vi "Compile - Tx Buffered Channel Refs.vi"(6 "Packet Name":string, 7 "Timestamp Present?":bool, 8 "error in (no error)":errorcluster, 11 "Item Ref in":T1 format="%.0x") -> (0 "error out":errorcluster, 3 "Item Ref out":T1 format="%.0x", 4 "Tx Ref Array":T2(array[cluster]) {"VS Refs" format="%.0x"})   [LabVIEW 2019, in "UDP-Custom-Device System Explorer.lvlib"]
uses:
  UDP-Custom-Device System Explorer.lvlib
  <vilib>/NI VeriStand/Custom Device API/Custom Device Item Ref.ctl
  Property Accessors/Tx Packet Accessors.lvlib
  <vilib>/NI VeriStand/Custom Device API/Custom Device API.lvlib
  Property Accessors/Buffered Data Packet.lvlib
  <vilib>/NI VeriStand/Custom Device Tools/Custom Device Utility Library/Custom Device Utility Library.lvlib
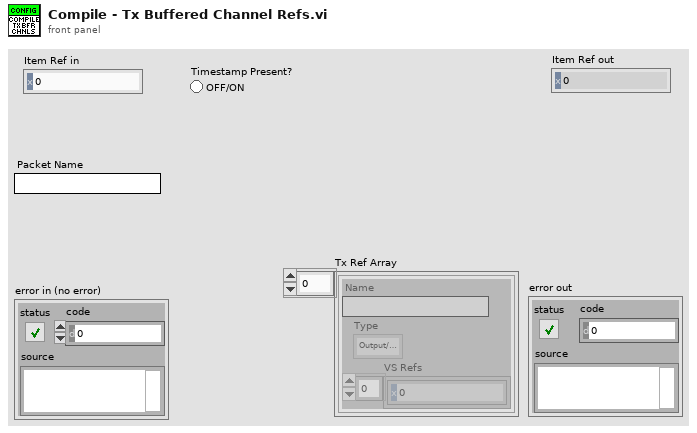
[diagram p1: front panel]
types:
  T1 = typedef "Custom Device API.lvlib/Custom Device Item Ref.ctl" = u64
  T2 = cluster{"Name":string, "Type":enum16{"Output/Write", "Input/Read", "Input/ReadWrite"}, "VS Refs":T1[]}[]
  T3 = cluster{"Name":string, "Type":enum16{"Output/Write", "Input/Read", "Input/ReadWrite"}, "VS Refs":T1[]}
  T4 = enum16{"Output/Write", "Input/Read", "Input/ReadWrite"}
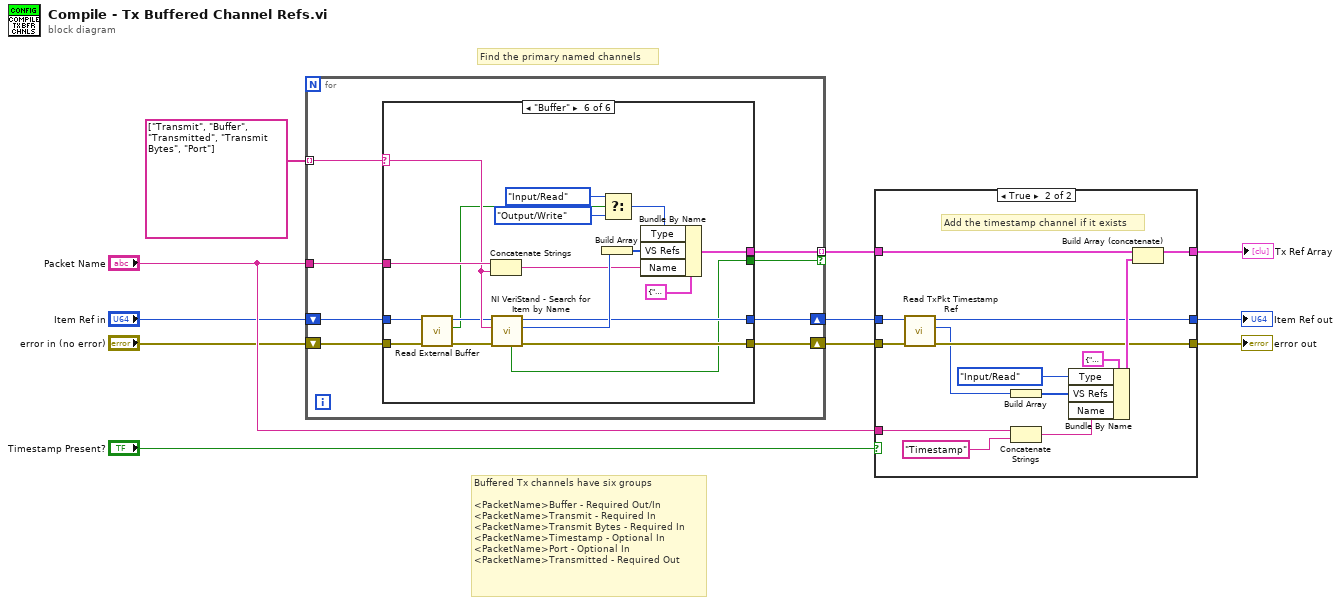
[diagram p0: block diagram]
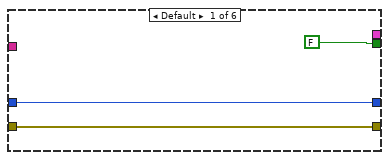
[diagram p3: hidden frame]
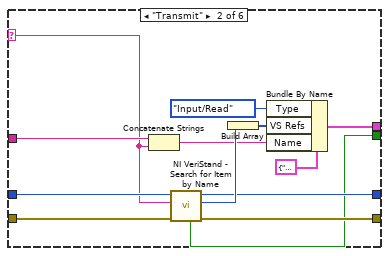
[diagram p4: hidden frame]
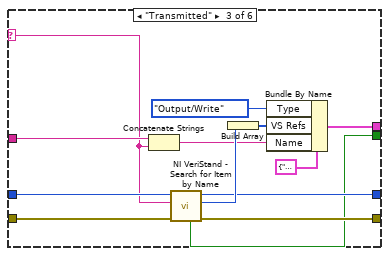
[diagram p5: hidden frame]
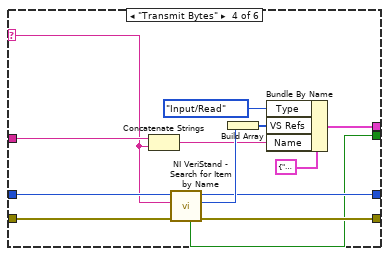
[diagram p6: hidden frame]
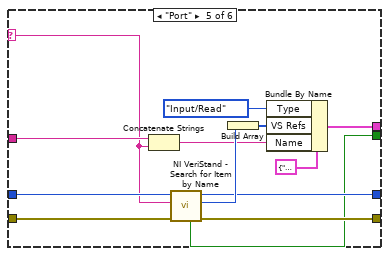
[diagram p7: hidden frame]
diagram:
  # "Find the primary named channels"
  # "Buffered Tx channels have six groups\n\n<PacketName>Buffer - Required Out/In\n<PacketName>Transmit - Required In\n<PacketName>Transmit Bytes - Required In\n<PacketName>Timestamp - Optional In\n<PacketName>Port - Optional In\n<PacketName>Transmitted - Required Out"
  n1 = for {
    tunnel: string[] ["Transmit", "Buffer", "Transmitted", "Transmit Bytes", "Port"] ("Item GUID") -> [w19] mode=indexing
    tunnel: "Packet Name" -> [w14]
    tunnel: [w16] -> w3 mode=indexing if=w15
    shift-right: [w13] -> w2
    shift-left: "Item Ref in" -> [w17]
    shift-right: [w12] -> w1
    shift-left: "error in (no error)" -> [w18]
    n2 = case shown="\"Buffer\"" w19 {
      selector: w19 -> [_ w24 w37 w50 w63 w84]
      tunnel: w18 -> [w21 w30 w43 w56 w69 w82]
      tunnel: w17 -> [w22 w31 w44 w57 w70 w80]
      tunnel: [w22 w29 w42 w55 w68 w89] -> w13
      tunnel: [w21 w28 w41 w54 w67 w88] -> w12
      tunnel: [_ w27 w40 w53 w66 w87] -> w16
      tunnel: [FALSE ("Found") w26 w39 w52 w65 w86] -> w15
      tunnel: w14 -> [_ w25 w38 w51 w64 w85]
      frame Default {
      }
      frame "Transmit" {
        n3 = Concatenate Strings(w25, w24) -> (w23:string)
        n4 = call <vilib>:"NI VeriStand - Search for Item by Name.vi"("error in"=w30, "Item Name"=w24, "Section Ref in"=w31) -> ("error out"=w28:errorcluster, "Item Ref"=w33:T1, "Section Ref out"=w29:T1, "Found"=w26:bool)  [unwired: 5 in]
        n5 = Build Array(w33) -> (w34:T1[])
        n6 = Bundle By Name(cluster=T3 {"Name"="", "Type"=enum."Output/Write", "VS Refs"=[]} ("Group"), "Type"=T4."Input/Read", "VS Refs"=w34, "Name"=w23) -> (w27:T3)
      }
      frame "Transmitted" {
        n7 = Concatenate Strings(w38, w37) -> (w36:string)
        n8 = call <vilib>:"NI VeriStand - Search for Item by Name.vi"("error in"=w43, "Item Name"=w37, "Section Ref in"=w44) -> ("error out"=w41:errorcluster, "Item Ref"=w46:T1, "Section Ref out"=w42:T1, "Found"=w39:bool)  [unwired: 5 in]
        n9 = Build Array(w46) -> (w47:T1[])
        n10 = Bundle By Name(cluster=T3 {"Name"="", "Type"=enum."Output/Write", "VS Refs"=[]} ("Group"), "Type"=T4."Output/Write", "VS Refs"=w47, "Name"=w36) -> (w40:T3)
      }
      frame "Transmit Bytes" {
        n11 = Concatenate Strings(w51, w50) -> (w49:string)
        n12 = call <vilib>:"NI VeriStand - Search for Item by Name.vi"("error in"=w56, "Item Name"=w50, "Section Ref in"=w57) -> ("error out"=w54:errorcluster, "Item Ref"=w59:T1, "Section Ref out"=w55:T1, "Found"=w52:bool)  [unwired: 5 in]
        n13 = Build Array(w59) -> (w60:T1[])
        n14 = Bundle By Name(cluster=T3 {"Name"="", "Type"=enum."Output/Write", "VS Refs"=[]} ("Group"), "Type"=T4."Input/Read", "VS Refs"=w60, "Name"=w49) -> (w53:T3)
      }
      frame "Port" {
        n15 = Concatenate Strings(w64, w63) -> (w62:string)
        n16 = call <vilib>:"NI VeriStand - Search for Item by Name.vi"("error in"=w69, "Item Name"=w63, "Section Ref in"=w70) -> ("error out"=w67:errorcluster, "Item Ref"=w72:T1, "Section Ref out"=w68:T1, "Found"=w65:bool)  [unwired: 5 in]
        n17 = Build Array(w72) -> (w73:T1[])
        n18 = Bundle By Name(cluster=T3 {"Name"="", "Type"=enum."Output/Write", "VS Refs"=[]} ("Group"), "Type"=T4."Input/Read", "VS Refs"=w73, "Name"=w62) -> (w66:T3)
      }
      frame "Buffer" {
        n19 = call "Read External Buffer.vi"("error in (no error)"=w82, "Node Ptr"=w80) -> ("error out"=w81:errorcluster, "External Buffer"=w76:bool, "Node Ptr out"=w79:T1)  [unwired: 7 in]
        n20 = Concatenate Strings(w85, w84) -> (w83:string)
        n21 = call <vilib>:"NI VeriStand - Search for Item by Name.vi"("error in"=w81, "Item Name"=w84, "Section Ref in"=w79) -> ("error out"=w88:errorcluster, "Item Ref"=w91:T1, "Section Ref out"=w89:T1, "Found"=w86:bool)  [unwired: 5 in]
        n22 = Build Array(w91) -> (w92:T1[])
        n23 = Select(t=T4."Input/Read" ("Type"), s=w76, f=T4."Output/Write" ("Type")) -> (s? t:f=w75:T4)
        n24 = Bundle By Name(cluster=T3 {"Name"="", "Type"=enum."Output/Write", "VS Refs"=[]} ("Group"), "Type"=w75, "VS Refs"=w92, "Name"=w83) -> (w87:T3)
      }
    }
  }
  n25 = case shown="True" "Timestamp Present?" {
    tunnel: w3 -> [w95 w109]
    tunnel: w2 -> [w94 w100]
    tunnel: [w94 w99] -> w9
    tunnel: [w93 w97] -> w8
    tunnel: w1 -> [w93 w98]
    tunnel: [w95 w108] -> w7
    tunnel: "Packet Name" -> [_ w101]
    frame False {
    }
    frame True {
      # "Add the timestamp channel if it exists"
      n26 = call "Read TxPkt Timestamp Ref.vi"("error in (no error)"=w98, "Node Ptr"=w100) -> ("error out"=w97:errorcluster, "Timestamp Ref"=w96:T1, "Node Ptr out"=w99:T1)  [unwired: 7 in]
      n27 = Build Array(w96) -> (w104:T1[])
      n28 = Concatenate Strings(w101, "Timestamp" ("Item GUID")) -> (w105:string)
      n29 = Bundle By Name(cluster=T3 {"Name"="", "Type"=enum."Output/Write", "VS Refs"=[]} ("Group"), "Type"=T4."Input/Read", "VS Refs"=w104, "Name"=w105) -> (w102:T3)
      n30 = Build Array (concatenate)(w109, w102) -> (w108:T2)
    }
  }
  "Tx Ref Array" <- w7
  "error out" <- w8
  "Item Ref out" <- w9
